vi "Calculate Freq Detuning.vi"() -> ()   [LabVIEW 2013]
panel:
  out "Freq Detuning":dbl[](array[numeric])
  out "Delta Freq(GHZ)":dbl
  in  "Central Wavelength":dbl=975.47
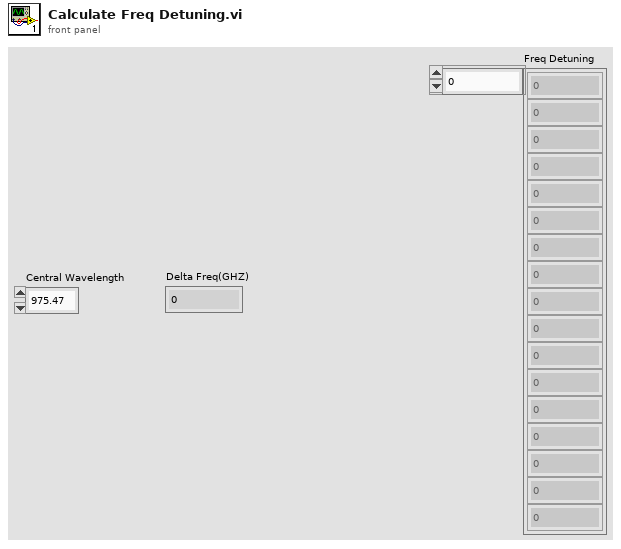
[diagram p1: front panel]
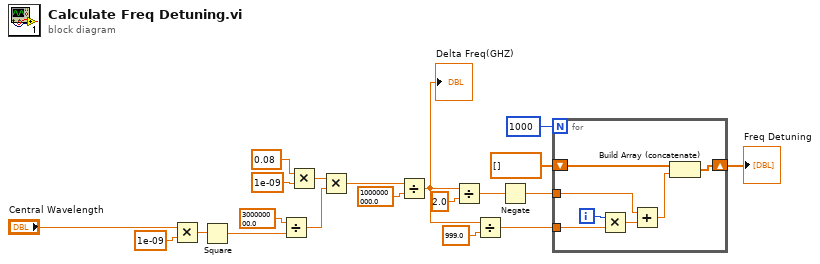
[diagram p0: block diagram]
diagram:
  n1 = Multiply(x="Central Wavelength", y=1e-09 ("x")) -> (x*y=w16:dbl)
  n2 = Square(x=w16) -> (x^2=w15:dbl)
  n3 = Divide(x=300000000.0, y=w15) -> (x/y=w14:dbl)
  n4 = Multiply(x=0.08, y=1e-09 ("x")) -> (x*y=w11:dbl)
  n5 = Multiply(x=w11, y=w14) -> (x*y=w10:dbl)
  n6 = Divide(x=w10, y=1000000000.0 ("x")) -> (x/y=w6:dbl)
  "Delta Freq(GHZ)" <- w6
  n7 = Divide(x=w6, y=2.0) -> (x/y=w4:dbl)
  n8 = Divide(x=w6, y=999.0) -> (x/y=w7:dbl)
  n9 = Negate(x=w4) -> (-x=w3:dbl)
  n10 = for {
    N: 1000 -> [_]
    shift-right: [w22] -> w1
    shift-left: dbl[] [] -> [w21]
    tunnel: w7 -> [w26]
    tunnel: w3 -> [w25]
    i -> [w27]
    n11 = Multiply(x=w27, y=w26) -> (x*y=w24:dbl)
    n12 = Add(x=w25, y=w24) -> (x+y=w23:dbl)
    n13 = Build Array (concatenate)(w21, w23) -> (w22:dbl[])
  }
  "Freq Detuning" <- w1
